vi "Get Data from RAM.vi"(8 "error in (no error)":errorcluster, 9 "End offset":u64, 10 "Start offset":u64, 11 "RP Communicator in":refnum<class "RP Communicator VISA.lvclass">) -> (0 "error out":errorcluster, 2 "data out":string, 3 "RP Communicator out":refnum<class "RP Communicator VISA.lvclass">)   [LabVIEW 2019, in "RP Communicator VISA.lvclass"]
uses:
  RP Communicator VISA.lvclass
  RP Command.ctl
  RP Communicator VISA.lvclass/RP Communicator VISA.ctl
  RP Write Command VISA.vi
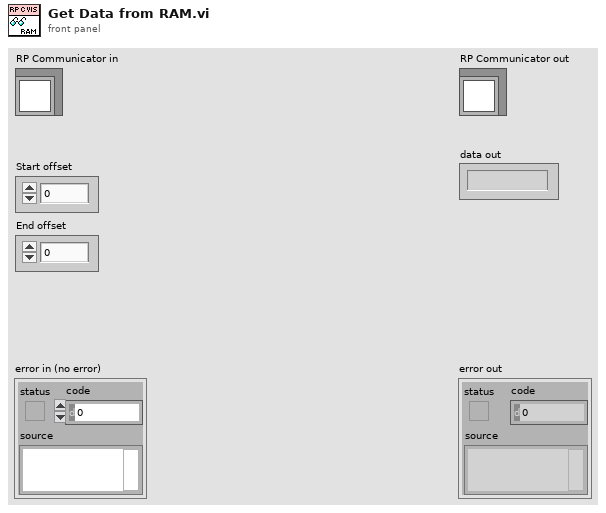
[diagram p1: front panel]
types:
  T1 = typedef "RP Command.ctl" = enum16{"Reset", "Read IDN", "Stop server", "Get status", "Get temperature", "Connect client", "Arm", "Software trigger", "Get whole buffer", "Get chunk", "System call", "Get config", "Set config", "Recieve data", "Recieve Calibartion", "Transmit data"}
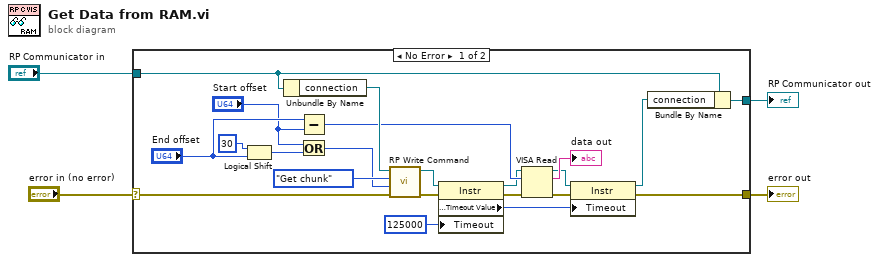
[diagram p0: block diagram]
diagram:
  n1 = case shown="No Error" "error in (no error)" {
    selector: "error in (no error)" -> [w16 w28]
    tunnel: [w5 w28] -> w3
    tunnel: [w17 w27] -> w1
    tunnel: "RP Communicator in" -> [w26 w27]
    frame No Error {
      n2 = Logical Shift(y=i16 30, x="End offset") -> (x << y=w22:u64)
      n3 = Unbundle By Name(w26) -> ("connection"=w25:refnum<visa-resource-name>)
      n4 = Subtract(x="End offset", y="Start offset") -> (x-y=w18:u64)
      n5 = Or(x="Start offset", y=w22) -> (x .or. y?=w21:u64)
      n6 = call-poly "RP Write Command.vi"("Error In"=w16, "Command payload"=w21, "Command number"=RP_Command."Get chunk", "VISA resource"=w25) -> ("Error Out"=w12:errorcluster, "VISA resource out"=w11:refnum<visa-resource-name>)  [unwired: 5 in, 1 out]
      n7 = property class="Instr"(reference=w11, error in=w12, "Timeout"=u32 125000 ("timeout ms (25000)")) -> (reference out=w9:refnum<visa-resource-name>, error out=w10:errorcluster, "General Settings:Timeout Value"=w14:u32)
      n8 = VISA Read(VISA resource name=w9, byte count=w18, error in (no error)=w10) -> (VISA resource name out=w8:refnum<visa-resource-name>, read buffer=→"data out":string, error out=w6:errorcluster)  [unwired: 1 out]
      n9 = property class="Instr"(reference=w8, error in=w6, "Timeout"=w14) -> (reference out=w7:refnum<visa-resource-name>, error out=w5:errorcluster)
      n10 = Bundle By Name(cluster=w26, "connection"=w7) -> (w17:refnum<class "RP Communicator VISA.lvclass">)
    }
    frame Error {
    }
  }
  "error out" <- w3
  "RP Communicator out" <- w1
